vi "hamamatsuReadAsync.vi"   [LabVIEW 2017]
doc: "Reads into disk the frames from the Hamamatsu camera. The frames are written to disk asynchronously from the \"Wait for next frame\" VI, to avoid frame drops.\n\nWhen this VI stops, it issues a daqStop to stop the acquisition from the DAQ card."
uses:
  globalDevices.vi
  globalUtilities.vi
types:
  T1 = enum16{"big-endian, network order", "native, host order", "little-endian"}
  T2 = enum16{"open", "replace", "create", "open or create", "replace or create", "replace or create with confirmation"}
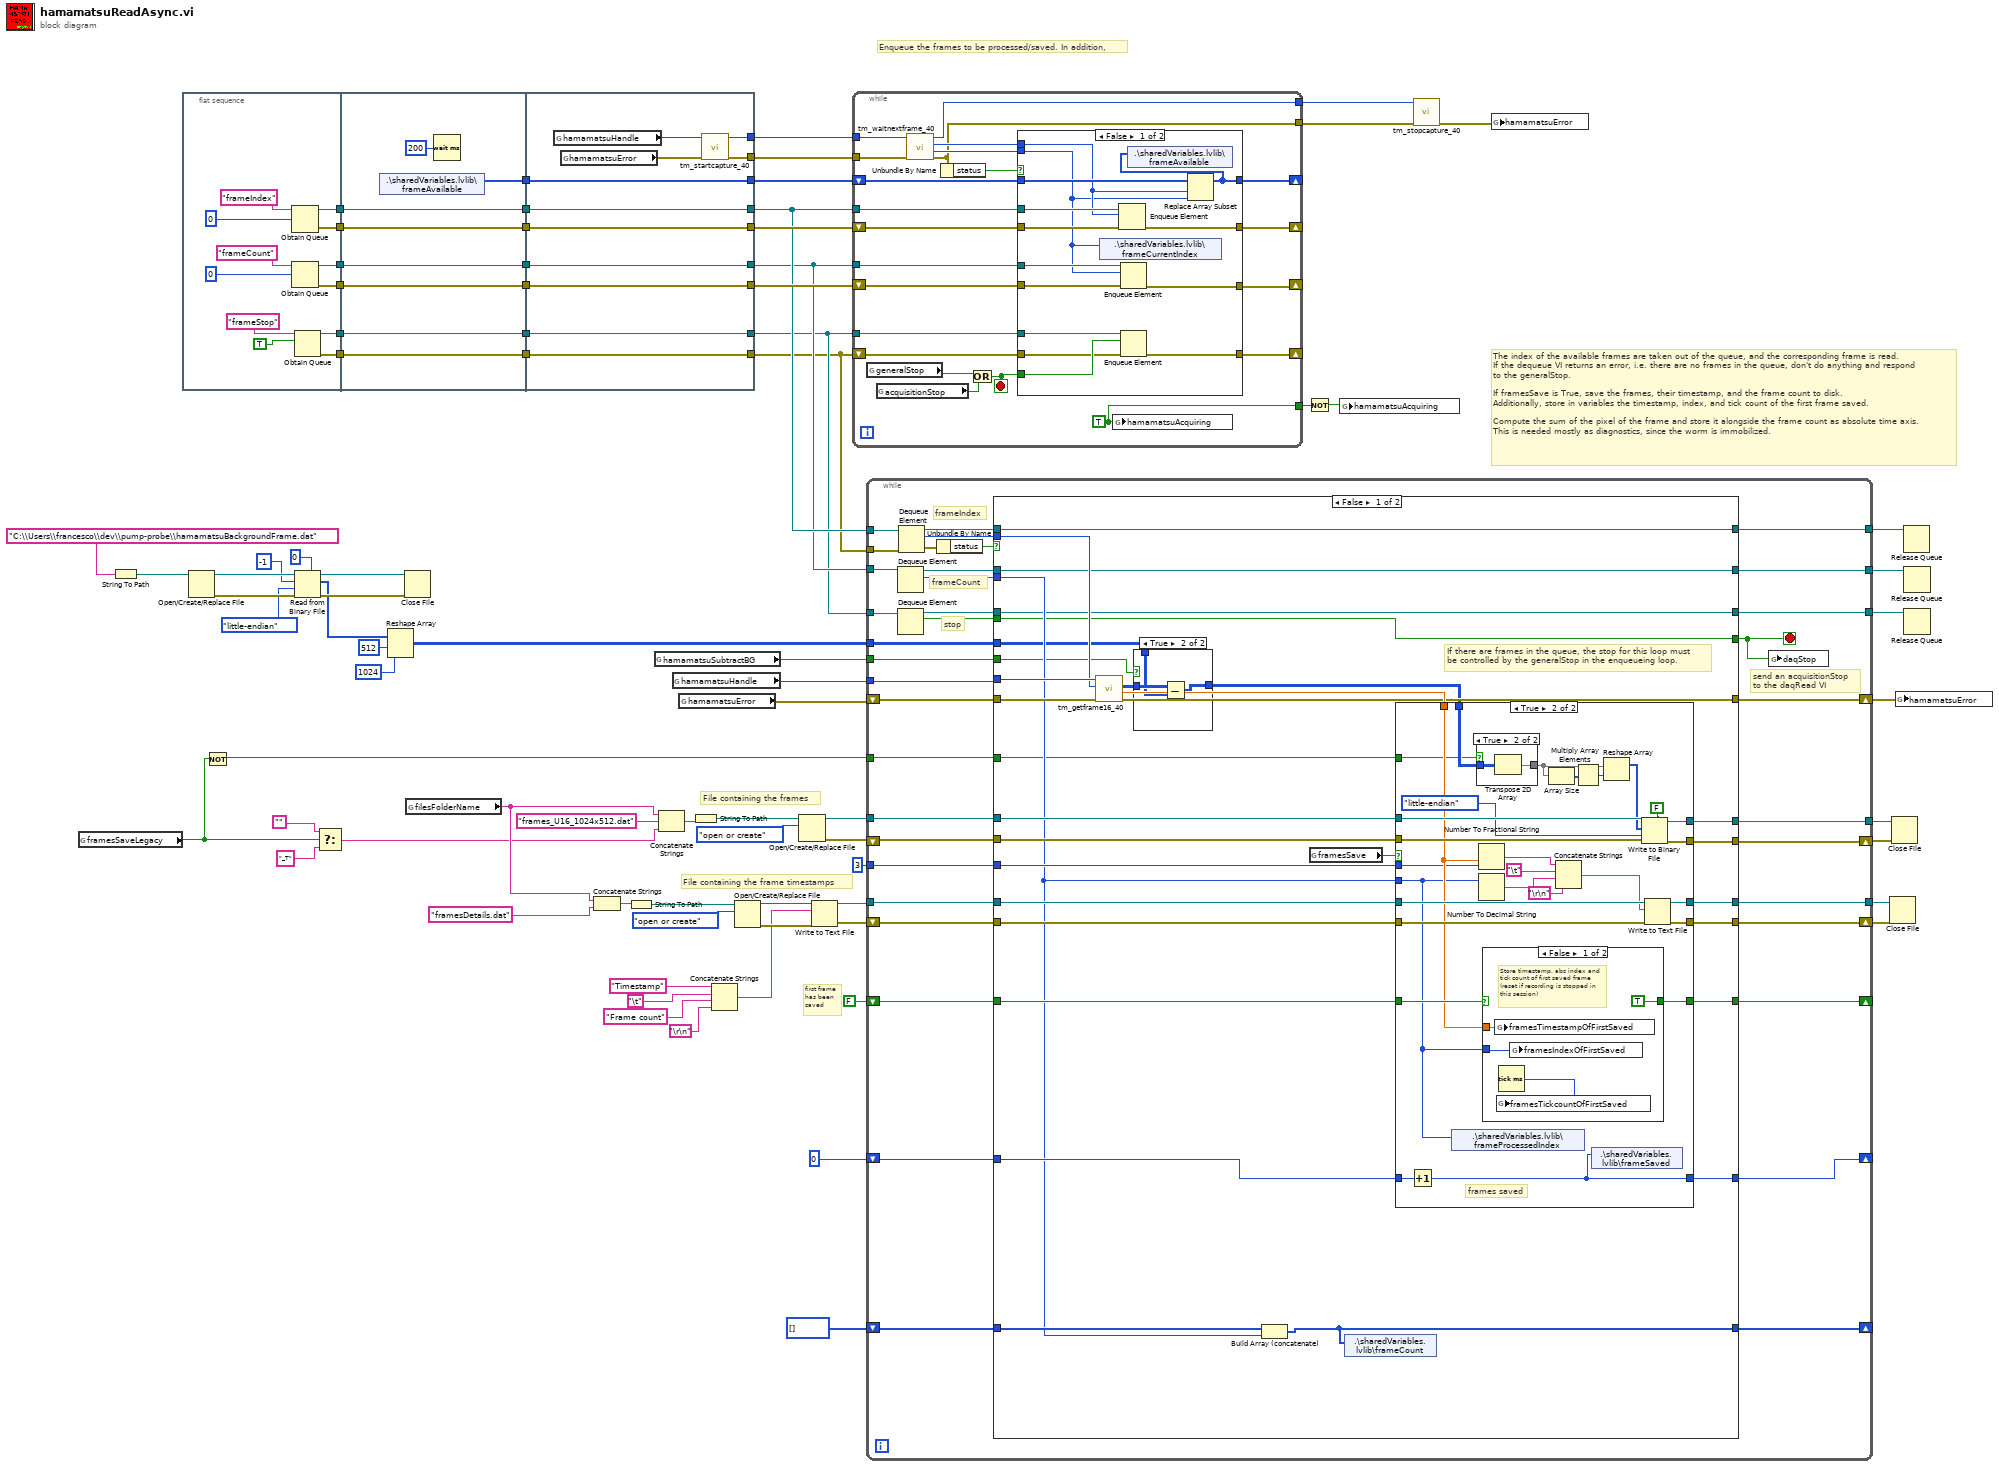
[diagram p0: block diagram]
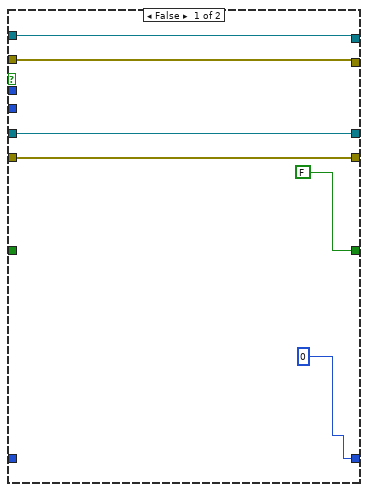
[diagram p3: hidden frame]
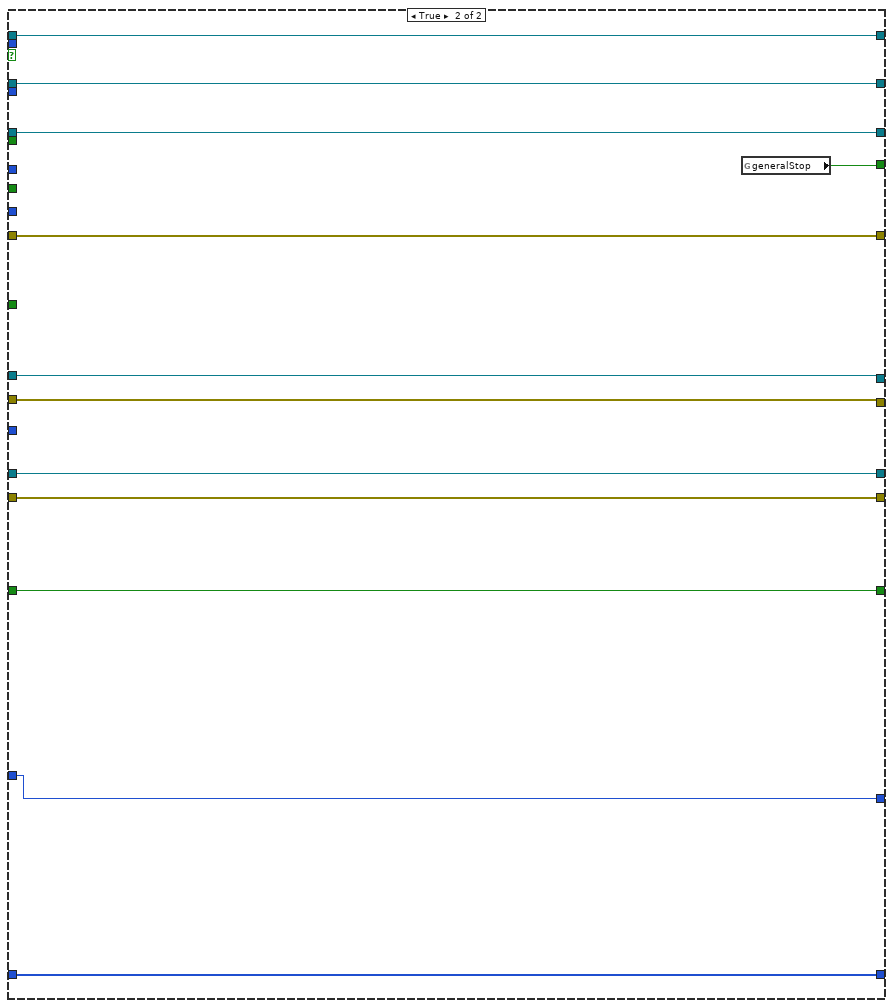
[diagram p6: hidden frame]
diagram:
  # "Enqueue the frames to be processed/saved. In addition,"
  # "first frame\nhas been\nsaved"
  # "The index of the available frames are taken out of the queue, and the corresponding frame is read.\nIf the dequeue VI returns an error, i.e. there are no frames in the queue, don't do anything and respond\nto the generalStop.\n\nIf framesSave is True, save the frames, their timestamp, and the frame count to disk.\nAdditionally, store in variables the timestamp, index, and tick count of the first frame saved.\n\nCompute the sum of the pixel of the frame and store it alongside the frame count as absolute time axis.\nThis is needed mostly as diagnostics, since the worm is immobilized."
  # "File containing the frame timestamps"
  # "File containing the frames"
  n1 = global read "globalUtilities.vi" "framesSaveLegacy"() -> (w2:bool)
  n2 = String To Path(string="C:\\Users\\francesco\\dev\\pump-probe\\hamamatsuBackgroundFrame.dat") -> (path=w23:path)
  n3 = flat-sequence {
    tunnel: [w88] -> w38
    tunnel: [w85] -> w36
    tunnel: [w84] -> w34
    tunnel: [w83] -> w32
    tunnel: [w82] -> w30
    tunnel: [w81] -> w28
    tunnel: w38 -> [w100]
    tunnel: [w100] -> w37
    tunnel: w36 -> [w99]
    tunnel: [w99] -> w35
    tunnel: w34 -> [w98]
    tunnel: [w98] -> w33
    tunnel: w32 -> [w97]
    tunnel: [w97] -> w31
    tunnel: w30 -> [w96]
    tunnel: [w96] -> w29
    tunnel: w28 -> [w95]
    tunnel: [w95] -> w27
    tunnel: [w93] -> w10
    tunnel: [w106] -> w53
    tunnel: [w107] -> w54
    tunnel: [w108] -> w55
    tunnel: [w109] -> w56
    tunnel: [w110] -> w57
    tunnel: [w111] -> w80
    tunnel: w37 -> [w111]
    tunnel: w35 -> [w110]
    tunnel: w33 -> [w109]
    tunnel: w31 -> [w108]
    tunnel: w29 -> [w107]
    tunnel: w27 -> [w106]
    tunnel: [w103] -> w40
    tunnel: [w102] -> w39
    tunnel: w10 -> [w101]
    tunnel: [w101] -> w9
    frame #0 {
      n4 = Obtain Queue(name (unnamed)="frameIndex", element data type=0) -> (queue out=w84:refnum<queue>, error out=w88:errorcluster)  [unwired: 3 in, 1 out]
      n5 = Obtain Queue(name (unnamed)="frameCount", element data type=0) -> (queue out=w83:refnum<queue>, error out=w85:errorcluster)  [unwired: 3 in, 1 out]
      n6 = Obtain Queue(name (unnamed)="frameStop", element data type=TRUE) -> (queue out=w82:refnum<queue>, error out=w81:errorcluster)  [unwired: 3 in, 1 out]
    }
    frame #1 {
      n7 = shared-variable ".\\sharedVariables.lvlib\\frameAvailable"() -> (w93:i32[])  [unwired: 1 in, 1 out]
      n8 = Wait (ms)(milliseconds to wait=u32 200) -> ()  [unwired: 1 out]
    }
    frame #2 {
      n9 = global read "globalDevices.vi" "hamamatsuHandle"() -> (w105:u32)
      n10 = global read "globalDevices.vi" "hamamatsuError"() -> (w104:errorcluster)
      n11 = call <userlib>:"tm_startcapture_40.vi"("error in (no error)"=w104, "Handle in"=w105) -> ("error out"=w103:errorcluster, "Handle out"=w102:u32)  [unwired: 8 in]
    }
  }
  n12 = Open/Create/Replace File(file path (use dialog)=w23) -> (refnum out=w22:refnum<file>, error out=w21:errorcluster)  [unwired: 5 in, 1 out]
  n13 = Not(x=w2) -> (.not. x?=w1:bool)
  n14 = Read from Binary File(5:u16 0, 8:w21, 9:T1."little-endian" ("byte order (0:big-endian, network order)"), 10:-1 ("count (1)"), 11:w22) -> (0:w16:errorcluster, 2:w15:u16[], 3:w17:refnum<file>)  [unwired: 1 in, 1 out]
  n15 = Select(t="", s=w2, f="_T") -> (s? t:f=w3:string)
  n16 = Reshape Array(w15, 512 ("dimension size"), 1024 ("dimension size")) -> (w11:u16[][])
  n17 = Close File(refnum=w17, error in=w16) -> ()  [unwired: 2 out]
  n18 = global read "globalUtilities.vi" "filesFolderName"() -> (w60:string)
  n19 = Concatenate Strings(w60, "framesDetails.dat") -> (w70:string)
  n20 = String To Path(string=w70) -> (path=w71:path)
  n21 = global read "globalDevices.vi" "hamamatsuSubtractBG"() -> (w12:bool)
  n22 = Concatenate Strings(w60, "frames_U16_1024x512.dat", w3) -> (w75:string)
  n23 = global read "globalDevices.vi" "hamamatsuHandle"() -> (w79:u32)
  n24 = global read "globalDevices.vi" "hamamatsuError"() -> (w78:errorcluster)
  n25 = String To Path(string=w75) -> (path=w74:path)
  n26 = Concatenate Strings("Timestamp", "\t", "Frame count", "\r\n") -> (w41:string)
  n27 = Open/Create/Replace File(file path (use dialog)=w71, operation (0:open)=T2."open or create") -> (refnum out=w65:refnum<file>, error out=w64:errorcluster)  [unwired: 4 in, 1 out]
  n28 = Open/Create/Replace File(file path (use dialog)=w74, operation (0:open)=T2."open or create") -> (refnum out=w73:refnum<file>, error out=w67:errorcluster)  [unwired: 4 in, 1 out]
  n29 = Write to Text File(file (use dialog)=w65, text=w41, error in=w64) -> (refnum out=w63:refnum<file>, error out=w62:errorcluster)  [unwired: 1 in, 1 out]
  n30 = while {
    tunnel: w56 -> [w132]
    tunnel: w54 -> [w130]
    tunnel: w55 -> [w127]
    shift-right: [w125] -> _
    shift-left: w80 -> [w131]
    shift-right: [w124] -> _
    shift-left: w57 -> [w128]
    shift-right: [w123] -> _
    shift-left: w53 -> [w129]
    tunnel: w40 -> [w121]
    tunnel: w39 -> [w120]
    tunnel: [w119] -> w26
    tunnel: [w118] -> w25
    shift-right: [w113] -> _
    shift-left: w9 -> [w114]
    tunnel: [w112] -> w8
    stop <- w117 stop-if-true
    w112 = TRUE ("hamamatsuAcquiring")
    n31 = global read "globalUtilities.vi" "generalStop"() -> (w116:bool)
    n32 = global read "globalUtilities.vi" "acquisitionStop"() -> (w115:bool)
    n33 = call <userlib>:"tm_waitnextframe_40.vi"("error in (no error)"=w121, "Handle in"=w120) -> ("error out"=w118:errorcluster, "Frame Count"=w126:i32, "Frame Index"=w133:i32, "Handle out"=w119:u32)  [unwired: 6 in]
    n34 = Unbundle By Name(w118) -> ("status"=w122:bool)
    n35 = Or(x=w116, y=w115) -> (x .or. y?=w117:bool)
    n36 = case shown="False" w122 {
      tunnel: w133 -> [w136 _]
      tunnel: w132 -> [w147 _]
      tunnel: w131 -> [w146 w151]
      tunnel: w130 -> [w145 _]
      tunnel: w117 -> [w144 _]
      tunnel: w129 -> [w143 w149]
      tunnel: w128 -> [w142 w150]
      tunnel: w127 -> [w141 _]
      tunnel: w126 -> [w134 _]
      tunnel: [w140 w151] -> w125
      tunnel: [w139 w150] -> w124
      tunnel: [w138 w149] -> w123
      tunnel: w114 -> [w137 w148]
      tunnel: [w135 w148] -> w113
      frame False {
        n37 = shared-variable ".\\sharedVariables.lvlib\\frameCurrentIndex"(w134) -> ()  [unwired: 1 in, 1 out]
        n38 = Enqueue Element(queue=w147, element=w136, error in (no error)=w146) -> (error out=w140:errorcluster)  [unwired: 1 in, 2 out]
        n39 = Enqueue Element(queue=w141, element=w134, error in (no error)=w142) -> (error out=w139:errorcluster)  [unwired: 1 in, 2 out]
        n40 = Enqueue Element(queue=w145, element=w144, error in (no error)=w143) -> (error out=w138:errorcluster)  [unwired: 1 in, 2 out]
        n41 = Replace Array Subset(array=w137, new element=w134, index=w136) -> (w135:i32[])
        n42 = shared-variable ".\\sharedVariables.lvlib\\frameAvailable"(w135) -> ()  [unwired: 1 in, 1 out]
      }
      frame True {
      }
    }
    n43 = global write "globalUtilities.vi" "hamamatsuAcquiring"(w112) -> ()
  }
  n44 = while {
    tunnel: w79 -> [w165]
    tunnel: w73 -> [w188]
    shift-right: [w181] -> _
    shift-left: FALSE -> [w182]
    tunnel: w63 -> [w187]
    shift-right: [w185] -> w47
    shift-left: w62 -> [w186]
    shift-right: [w183] -> w48
    shift-left: w67 -> [w184]
    tunnel: i16 3 ("precision (6)") -> [w180]
    shift-right: [w179] -> w61
    shift-left: w78 -> [w164]
    shift-right: [w177] -> _
    shift-left: i32[] [] -> [w178]
    shift-right: [w175] -> _
    shift-left: u32 0 -> [w176]
    tunnel: w56 -> [w174]
    tunnel: w55 -> [w170]
    tunnel: w54 -> [w168]
    tunnel: w53 -> [w166]
    tunnel: [w162] -> w50
    tunnel: [w160] -> w51
    tunnel: [w158] -> w52
    tunnel: [w157] -> w49
    tunnel: [w156] -> w46
    tunnel: w12 -> [w154]
    tunnel: w11 -> [w153]
    tunnel: w1 -> [w152]
    stop <- w155 stop-if-true
    # "send an acquisitionStop\nto the daqRead VI"
    # "stop"
    # "frameCount"
    # "frameIndex"
    n45 = Dequeue Element(queue=w170) -> (queue out=w161:refnum<queue>, element=w169:i32)  [unwired: 2 in, 2 out]
    n46 = Dequeue Element(queue=w168) -> (queue out=w163:refnum<queue>, element=w167:bool)  [unwired: 2 in, 2 out]
    n47 = Dequeue Element(queue=w174, error in (no error)=w166) -> (queue out=w159:refnum<queue>, element=w171:i32, error out=w173:errorcluster)  [unwired: 1 in, 1 out]
    n48 = Unbundle By Name(w173) -> ("status"=w172:bool)
    n49 = case shown="False" w172 {
      tunnel: w164 -> [w219 w276]
      tunnel: w165 -> [w218 _]
      tunnel: w188 -> [w217 w267]
      tunnel: w187 -> [w216 w266]
      tunnel: w186 -> [w215 w274]
      tunnel: [w214 w274] -> w185
      tunnel: w184 -> [w213 w275]
      tunnel: [w212 w275] -> w183
      tunnel: w182 -> [w209 w273]
      tunnel: [w208 w273] -> w181
      tunnel: w180 -> [w207 _]
      tunnel: [w206 w276] -> w179
      tunnel: w178 -> [w205 w271]
      tunnel: [w204 w271] -> w177
      tunnel: w176 -> [w203 w272]
      tunnel: [w202 w272] -> w175
      tunnel: w171 -> [w201 _]
      tunnel: w169 -> [w200 _]
      tunnel: w167 -> [w199 _]
      tunnel: [w199 w277] -> w155
      tunnel: w163 -> [w198 w268]
      tunnel: [w198 w268] -> w162
      tunnel: w161 -> [w197 w269]
      tunnel: [w197 w269] -> w160
      tunnel: w159 -> [w196 w270]
      tunnel: [w196 w270] -> w158
      tunnel: [w195 w267] -> w157
      tunnel: [w194 w266] -> w156
      tunnel: w154 -> [w193 _]
      tunnel: w153 -> [w190 _]
      tunnel: w152 -> [w189 _]
      frame False {
        # "If there are frames in the queue, the stop for this loop must\nbe controlled by the generalStop in the enqueueing loop."
        n50 = call <userlib>:"tm_getframe16_40.vi"("error in (no error)"=w219, "Frame Index"=w201, "Handle in"=w218) -> ("error out"=w206:errorcluster, "Timestamp"=w210:dbl, "Data"=w192:u16[][])  [unwired: 5 in, 1 out]
        n51 = case shown="True" w193 {
          tunnel: w192 -> [w220 w223]
          tunnel: [w220 w221] -> w191
          tunnel: w190 -> [_ w222]
          frame False {
          }
          frame True {
            n52 = Subtract(x=w223, y=w222) -> (x-y=w221:u16[][])
          }
        }
        n53 = Build Array (concatenate)(w205, w200) -> (w204:i32[])
        n54 = global read "globalUtilities.vi" "framesSave"() -> (w211:bool)
        n55 = shared-variable ".\\sharedVariables.lvlib\\frameCount"(w204) -> ()  [unwired: 1 in, 1 out]
        n56 = case shown="True" w211 {
          tunnel: w217 -> [w225 w257]
          tunnel: w191 -> [_ w255]
          tunnel: w216 -> [w224 w253]
          tunnel: w210 -> [_ w246]
          tunnel: w215 -> [w228 w252]
          tunnel: [w228 w251] -> w214
          tunnel: w213 -> [w229 w250]
          tunnel: [w229 w249] -> w212
          tunnel: w209 -> [_ w248]
          tunnel: [FALSE w247] -> w208
          tunnel: w200 -> [_ w237]
          tunnel: w207 -> [_ w245]
          tunnel: w203 -> [_ w241]
          tunnel: [u32 0 w238] -> w202
          tunnel: [w225 w240] -> w195
          tunnel: [w224 w239] -> w194
          tunnel: w189 -> [_ w230]
          frame False {
          }
          frame True {
            # "frames saved"
            n57 = Increment(x=w241) -> (x+1=w238:u32)
            n58 = shared-variable ".\\sharedVariables.lvlib\\frameProcessedIndex"(w237) -> ()  [unwired: 1 in, 1 out]
            n59 = case shown="True" w230 {
              tunnel: w255 -> [w258 w260]
              tunnel: [w258 w259] -> w233
              frame False {
              }
              frame True {
                n60 = Transpose 2D Array(2D array=w260) -> (transposed array=w259:u16[][])
              }
            }
            n61 = Number To Fractional String(number=w246, precision (6)=w245) -> (F-format string=w244:string)  [unwired: 2 in]
            n62 = Number To Decimal String(number=w237) -> (decimal integer string=w243:string)  [unwired: 1 in]
            n63 = case shown="False" w248 {
              selector: w248 -> [_ w265]
              tunnel: [TRUE w265] -> w247
              tunnel: w246 -> [w263 _]
              tunnel: w237 -> [w262 _]
              frame False {
                # "Store timestamp, abs index and\ntick count of first saved frame\n(reset if recording is stopped in\nthis session)"
                n64 = global write "globalUtilities.vi" "framesTimestampOfFirstSaved"(w263) -> ()
                n65 = Tick Count (ms)() -> (millisecond timer value=w261:u32)
                n66 = global write "globalUtilities.vi" "framesTickcountOfFirstSaved"(w261) -> ()
                n67 = global write "globalUtilities.vi" "framesIndexOfFirstSaved"(w262) -> ()
              }
              frame True {
              }
            }
            n68 = Array Size(array=w233) -> (size(s)=w232:i32[])
            n69 = Concatenate Strings(w244, "\t", w243, "\r\n") -> (w242:string)
            n70 = Multiply Array Elements(1:w232) -> (0:w231:i32)
            n71 = shared-variable ".\\sharedVariables.lvlib\\frameSaved"(w238) -> ()  [unwired: 1 in, 1 out]
            n72 = Reshape Array(w233, w231) -> (w234:u16[])
            n73 = Write to Binary File(file (use dialog)=w257, data=w234, error in=w250, 5:FALSE ("prepend array or string size? (T)"), 9:T1."little-endian" ("byte order (0:big-endian, network order)")) -> (refnum out=w240:refnum<file>, error out=w249:errorcluster)  [unwired: 1 in, 1 out]
            n74 = Write to Text File(file (use dialog)=w253, text=w242, error in=w252) -> (refnum out=w239:refnum<file>, error out=w251:errorcluster)  [unwired: 1 in, 1 out]
          }
        }
      }
      frame True {
        n75 = global read "globalUtilities.vi" "generalStop"() -> (w277:bool)
      }
    }
    n76 = global write "globalUtilities.vi" "daqStop"(w155) -> ()
  }
  n77 = Not(x=w8) -> (.not. x?=w7:bool)
  n78 = global write "globalUtilities.vi" "hamamatsuAcquiring"(w7) -> ()
  n79 = call <userlib>:"tm_stopcapture_40.vi"("error in (no error)"=w25, "Handle in"=w26) -> ("error out"=w6:errorcluster)  [unwired: 8 in, 1 out]
  n80 = global write "globalDevices.vi" "hamamatsuError"(w6) -> ()
  n81 = Close File(refnum=w46, error in=w47) -> ()  [unwired: 2 out]
  n82 = Close File(refnum=w49, error in=w48) -> ()  [unwired: 2 out]
  n83 = global write "globalDevices.vi" "hamamatsuError"(w61) -> ()
  n84 = Release Queue(queue=w52) -> ()  [unwired: 2 in, 3 out]
  n85 = Release Queue(queue=w51) -> ()  [unwired: 2 in, 3 out]
  n86 = Release Queue(queue=w50) -> ()  [unwired: 2 in, 3 out]
